vi "Update Digital Config.vi"(8 "error in (no error)":errorcluster, 11 "Señal Digital":T1={"Puertos/Pines"="", "Puerto"="DAQSim1", "Pines"=[], "Tiempo de AQ"=0.0, "Tiempo entre AQ"=0.0}) -> (0 "error out":errorcluster)   [LabVIEW 2020, in "Settings.lvlib"]
uses:
  Settings.lvlib
  Aqcisition/Digital Signal Config.ctl
  <vilib>/drjdpowell/SQLite Library/SQL Connection/Open (path).vi
  <vilib>/drjdpowell/SQLite Library/SQL Connection/Open (string).vi
  <vilib>/AdvancedString/Path To Command Line String.vi
  <vilib>/drjdpowell/SQLite Library/SQL Connection/Execute SQL (No results).vi
  <vilib>/drjdpowell/SQLite Library/SQL Connection/Connection.lvclass
  <vilib>/drjdpowell/SQLite Library/SQLite.lvlib
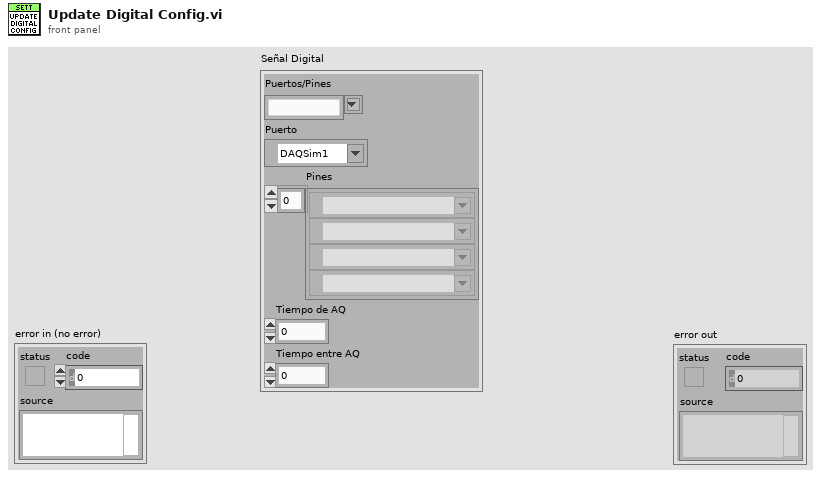
[diagram p1: front panel]
types:
  T1 = typedef "Digital Signal Config.ctl" = cluster{"Puertos/Pines":string, "Puerto":tag, "Pines":tag[], "Tiempo de AQ":dbl, "Tiempo entre AQ":dbl}
  T2 = cluster{"Pines[0]":tag, "Pines[1]":tag, "Pines[2]":tag, "Pines[3]":tag, "Pines[4]":tag, "Pines[5]":tag, "Pines[6]":tag, "Pines[7]":tag, "Pines[8]":tag}
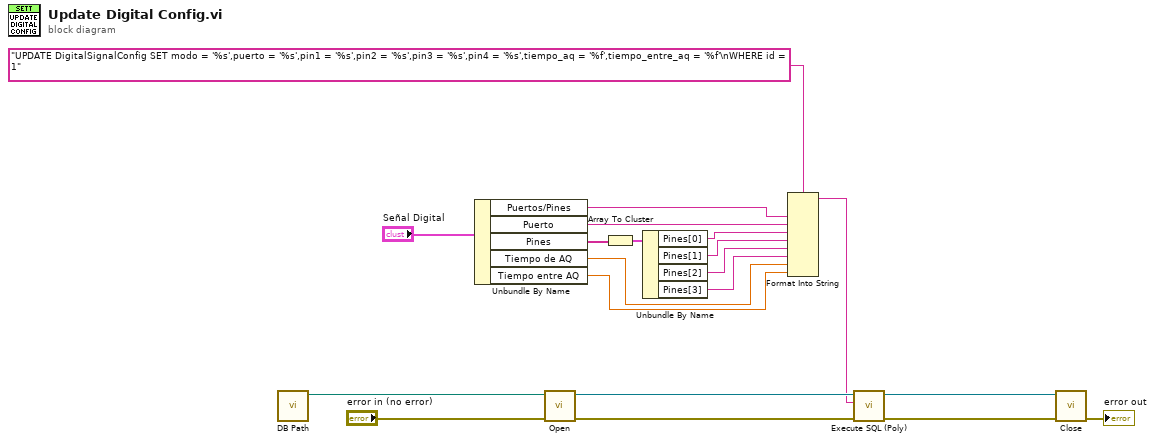
[diagram p0: block diagram]
diagram:
  n1 = call "DB Path.vi"() -> ("appended path"=w14:path)  [unwired: 11 in]
  n2 = Unbundle By Name("Señal Digital") -> ("Puertos/Pines"=w12:string, "Puerto"=w11:tag, "Pines"=w8:tag[], "Tiempo de AQ"=w2:dbl, "Tiempo entre AQ"=w1:dbl)
  n3 = call-poly <vilib>:"Open.vi"("error in (no error)"="error in (no error)", "db file"=w14) -> ("error out"=w20:errorcluster, "SQLite Connection"=w19:refnum<class "Connection.lvclass">)  [unwired: 8 in]
  n4 = Array To Cluster(array=w8) -> (cluster=w7:T2)
  n5 = Unbundle By Name(w7) -> ("Pines[0]"=w6:tag, "Pines[1]"=w5:tag, "Pines[2]"=w4:tag, "Pines[3]"=w3:tag)
  n6 = Format Into String(format string="UPDATE DigitalSignalConfig SET modo = '%s',puerto = '%s',pin1 = '%s',pin2 = '%s',pin3 = '%s',pin4 = '%s',tiempo_aq = '%f',tiempo_entre_aq = '%f'\nWHERE id = 1", w12, w11, w6, w5, w4, w3, w2, w1) -> (resulting string=w10:string)  [unwired: 2 in, 1 out]
  n7 = call-poly <vilib>:"Execute SQL (Poly).vi"("error in (no error)"=w20, "SQL"=w10, "SQLite Connection in"=w19) -> ("error out"=w18:errorcluster, "SQLite Connection"=w17:refnum<class "Connection.lvclass">)  [unwired: 7 in]
  n8 = call-dynamic "Close.vi"("error in (no error)"=w18, "SQLite Connection in"=w17) -> ("error out"=→"error out":errorcluster)  [unwired: 9 in]
